vi "Read NumberOfRobots.vi"(8 "error in (no error)":errorcluster, 11 "GoalKickAllyPlayVSS in":refnum<class "GoalKickAllyPlayVSS.lvclass">) -> (0 "error out":errorcluster, 2 "NumberOfRobots":dbl, 3 "GoalKickAllyPlayVSS out":refnum<class "GoalKickAllyPlayVSS.lvclass">)   [LabVIEW 2020, in "GoalKickAllyPlayVSS.lvclass"]
uses:
  GoalKickAllyPlayVSS.lvclass
  GoalKickAllyPlayVSS.lvclass/GoalKickAllyPlayVSS.ctl
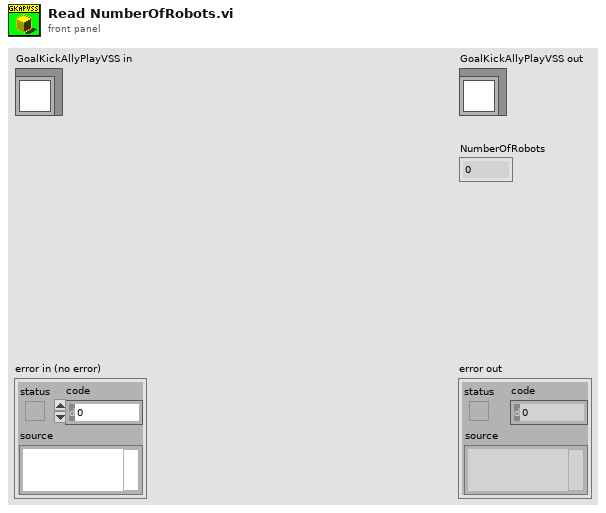
[diagram p1: front panel]
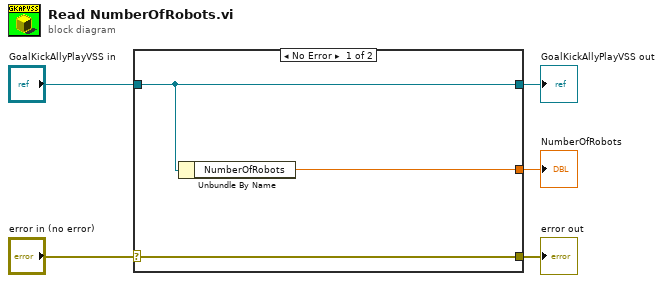
[diagram p0: block diagram]
diagram:
  n1 = case shown="No Error" "error in (no error)" {
    selector: "error in (no error)" -> [w8 w9]
    tunnel: [w8 w9] -> w4
    tunnel: [w7 w10] -> w2
    tunnel: "GoalKickAllyPlayVSS in" -> [w7 w10]
    tunnel: [w6 _] -> w1
    frame No Error {
      n2 = Unbundle By Name(w7) -> ("NumberOfRobots"=w6:dbl)
    }
    frame Error {
    }
  }
  "error out" <- w4
  "GoalKickAllyPlayVSS out" <- w2
  "NumberOfRobots" <- w1
